vi "Initialize.vi"(7 "Process ID":string, 8 "error in (no error)":errorcluster, 11 "STS Process in":refnum<class "STS Process.lvclass">) -> (0 "error out":errorcluster, 3 "STS Process out":refnum<class "STS Process.lvclass">)   [LabVIEW 2019, in "TimingDRV Engine.lvlib" / "STS Process.lvclass"]
uses:
  STS Process.lvclass
  C:/Users/nitest/Desktop/CD Project Tools/Source/Engine/Parent Classes/Process/Process.lvclass
  Parent Classes/Process/Process.lvclass/Process.ctl
  STS Process.lvclass/STS Process.ctl
  <vilib>/NI VeriStand/Custom Device API/Get Item Property (I32).vi
  <vilib>/NI VeriStand/Custom Device API/Get Item Property (Double).vi
  Parent Classes/Process/Process.lvclass
  <vilib>/NI VeriStand/Custom Device API/Custom Device API.lvlib
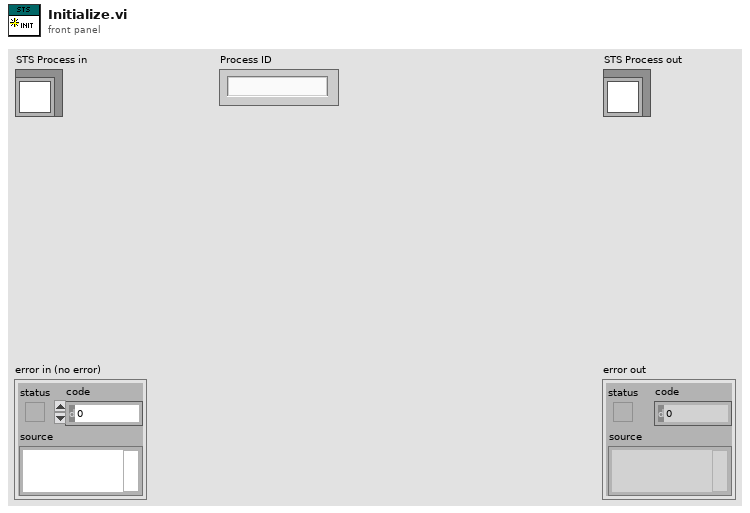
[diagram p1: front panel]
types:
  T1 = typedef "TimingDRV Engine.lvlib/Process.lvclass/Async Paramters.ctl" = cluster{"Device Reference":T2, "Device Clock":string, "Device Inputs FIFO":refnum<k33>, "Device Outputs FIFO":refnum<k33>, "CD Engine Event Ref":T3}
  T2 = typedef "Custom Device API.lvlib/Custom Device Item Ref.ctl" = u64
  T3 = typedef "Custom Device API.lvlib/Custom Device Engine Event Ref.ctl" = refnum<event-registration>
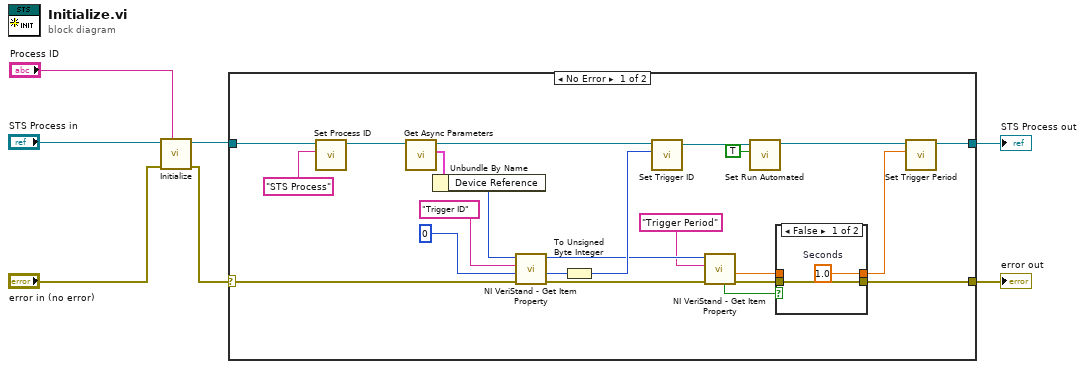
[diagram p0: block diagram]
diagram:
  n1 = call-parent "Initialize.vi"("Process ID"="Process ID", "error in (no error)"="error in (no error)", "Process in"="STS Process in") -> ("error out"=w3:errorcluster, "Process out"=w4:refnum<class "STS Process.lvclass">)  [unwired: 7 in]
  n2 = case shown="No Error" w3 {
    selector: w3 -> [w25 w35]
    tunnel: w4 -> [w14 w36]
    tunnel: [w10 w36] -> w2
    tunnel: [w8 w35] -> w1
    frame No Error {
      n3 = call "Set Process ID.vi"("Process ID"="STS Process", "CD_Process in"=w14) -> ("CD_Process out"=w13:refnum<class "STS Process.lvclass">)  [unwired: 9 in]
      n4 = call "Get Async Parameters.vi"("Process in"=w13) -> ("Async Parameters"=w30:T1, "Process out"=w24:refnum<class "STS Process.lvclass">)  [unwired: 9 in]
      n5 = Unbundle By Name(w30) -> ("Device Reference"=w26:T2)
      n6 = call-poly <vilib>:"NI VeriStand - Get Item Property.vi"("error in (no error)"=w25, "Default Value"=0, "Property Name"="Trigger ID", "Item Ref in"=w26) -> ("error out"=w20:errorcluster, "Value"=w27:i32, "Item Ref out"=w21:T2)  [unwired: 4 in, 1 out]
      n7 = To Unsigned Byte Integer(number=w27) -> (unsigned 8bit integer=w23:u8)
      n8 = call "Set Trigger ID.vi"("Trigger ID"=w23, "STS Process in"=w24) -> ("STS Process out"=w12:refnum<class "STS Process.lvclass">)  [unwired: 9 in]
      n9 = call-poly <vilib>:"NI VeriStand - Get Item Property.vi"("error in (no error)"=w20, "Property Name"="Trigger Period", "Item Ref in"=w21) -> ("error out"=w17:errorcluster, "Value"=w16:dbl, "Found?"=w18:bool)  [unwired: 5 in, 1 out]
      n10 = call "Set Run Automated.vi"("Run Automated"=TRUE, "STS Process in"=w12) -> ("STS Process out"=w11:refnum<class "STS Process.lvclass">)  [unwired: 9 in]
      n11 = case shown="False" w18 {
        tunnel: w17 -> [w31 w33]
        tunnel: w16 -> [_ w34]
        tunnel: [w32 w34] -> w9
        tunnel: [w31 w33] -> w8
        frame False {
          w32 = 1.0  # Seconds
        }
        frame True {
        }
      }
      n12 = call "Set Trigger Period.vi"("Trigger Period"=w9, "STS Process in"=w11) -> ("STS Process out"=w10:refnum<class "STS Process.lvclass">)  [unwired: 9 in]
    }
    frame Error {
    }
  }
  "error out" <- w1
  "STS Process out" <- w2
